vi "PicoScopeospaSetRapidSegments.vi"(5 "RapidBlock":bool=TRUE, 7 "nSegments":u64 format="%.4p", 8 "error in (no error)":errorcluster, 11 "handle in":i16) -> (0 "error out":errorcluster, 3 "handle out":i16, 6 "nCaptures":u64)   [LabVIEW 2010]
doc: "Calls SetDataBuffers, and assigns Pico buffers"
uses:
  psospa.dll
panel:
  out "nMaxSamples":u64
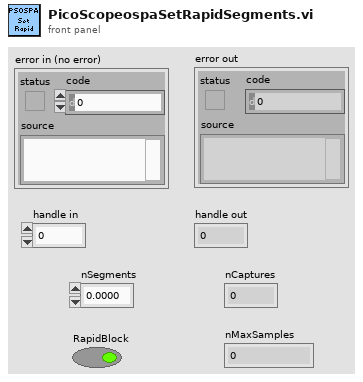
[diagram p1: front panel]
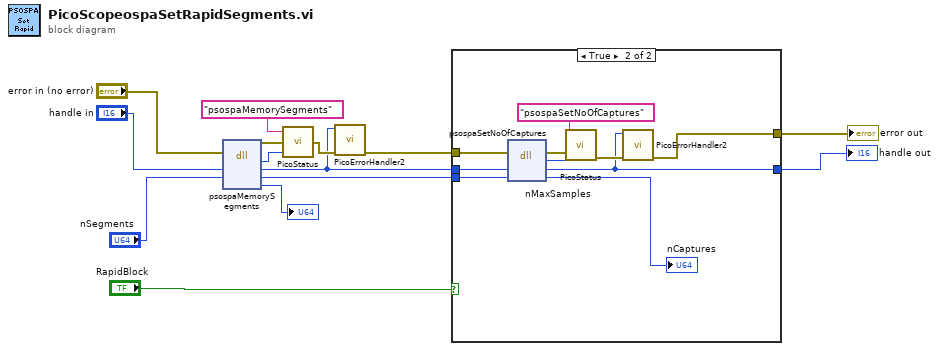
[diagram p0: block diagram]
diagram:
  n1 = dll-call lib="psospa.dll" fn="psospaMemorySegments" ("ps3000.dll:_ps3000_open_unit@0")(error in="error in (no error)", "handle"="handle in", "nSegments"="nSegments") -> (error out=w13:errorcluster, "PICO_STATUS"=w14:u32, "handle"=w9:i16, "nSegments"=w11:u64, "nMaxSamples"=→"nMaxSamples":u64)  [unwired: 3 in, 1 out]
  n2 = call "PicoStatus.vi"("PICO STATUS"=w14, "error in"=w13, "source"="psospaMemorySegments") -> ("error out"=w10:errorcluster)
  n3 = call "PicoErrorHandler2.vi"("error in (no error)"=w10, "handle In"=w9) -> ("error out"=w7:errorcluster)  [unwired: 9 in]
  n4 = case shown="True" "RapidBlock" {
    tunnel: w11 -> [_ w26]
    tunnel: w9 -> [w15 w23]
    tunnel: w7 -> [w16 w20]
    tunnel: [w16 w19] -> w4
    tunnel: [w15 w18] -> w3
    frame False {
    }
    frame True {
      n5 = dll-call lib="psospa.dll" fn="psospaSetNoOfCaptures" ("ps3000.dll:_ps3000_open_unit@0")(error in=w20, "handle"=w23, "nCaptures"=w26) -> (error out=w25:errorcluster, "PICO_STATUS"=w21:u32, "handle"=w18:i16, "nCaptures"=→"nCaptures":u64)  [unwired: 2 in, 1 out]
      n6 = call "PicoStatus.vi"("PICO STATUS"=w21, "error in"=w25, "source"="psospaSetNoOfCaptures") -> ("error out"=w22:errorcluster)
      n7 = call "PicoErrorHandler2.vi"("error in (no error)"=w22, "handle In"=w18) -> ("error out"=w19:errorcluster)  [unwired: 9 in]
    }
  }
  "error out" <- w4
  "handle out" <- w3
